vi "Write Name.vi"(8 "error in (no error)":errorcluster, 10 "Name":string, 11 "bt_Send_Queue in":refnum<class "bt_Send_Notifier.lvclass">) -> (0 "error out":errorcluster, 3 "bt_Send_Queue out":refnum<class "bt_Send_Notifier.lvclass">)   [LabVIEW 2021, in "BT.lvlib" / "bt_Send_Notifier.lvclass"]
uses:
  bt_Send_Notifier.lvclass
  bt_Send_Notifier.lvclass/bt_Send_Notifier.ctl
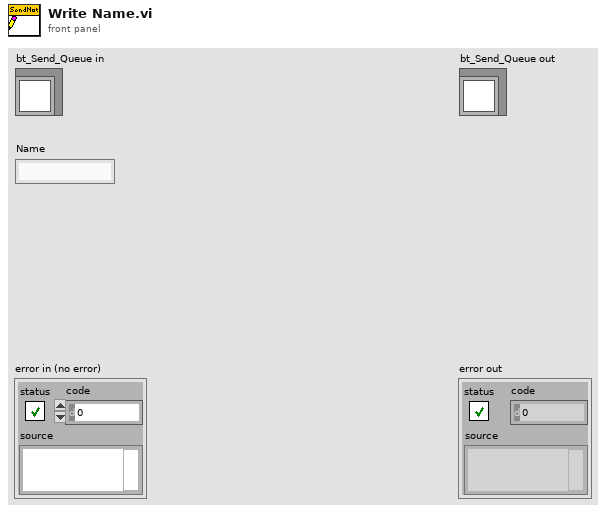
[diagram p1: front panel]
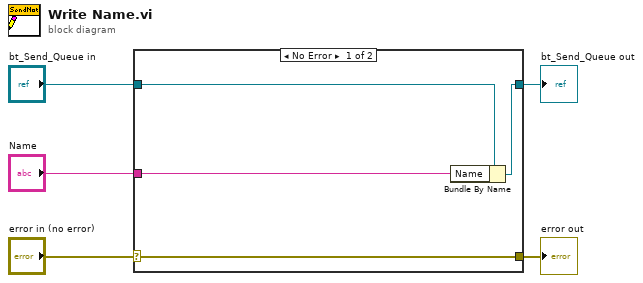
[diagram p0: block diagram]
diagram:
  n1 = case shown="No Error" "error in (no error)" {
    selector: "error in (no error)" -> [w9 w10]
    tunnel: [w9 w10] -> w4
    tunnel: [w7 w11] -> w2
    tunnel: "bt_Send_Queue in" -> [w8 w11]
    tunnel: "Name" -> [w6 _]
    frame No Error {
      n2 = Bundle By Name(cluster=w8, "Name"=w6) -> (w7:refnum<class "bt_Send_Notifier.lvclass">)
    }
    frame Error {
    }
  }
  "error out" <- w4
  "bt_Send_Queue out" <- w2
